vi "Plot Editor_Store to Plot.vi"(7 "XYGraph in":refnum<vi>, 8 "Error In":errorcluster, 11 "Plot Editor Internal Data":T1) -> (0 "Error Out":errorcluster, 3 "Plot Editor Internal Data (dup)":T1)   [LabVIEW 2021, in "Plot Editor.lvlib"]
uses:
  Plot Editor.lvlib
  Plot Editor Internal Variables.ctl
  XY Graph/XY Graph Plot Properties.ctl
  XY Graph/XY Graph Add-Ons.lvlib
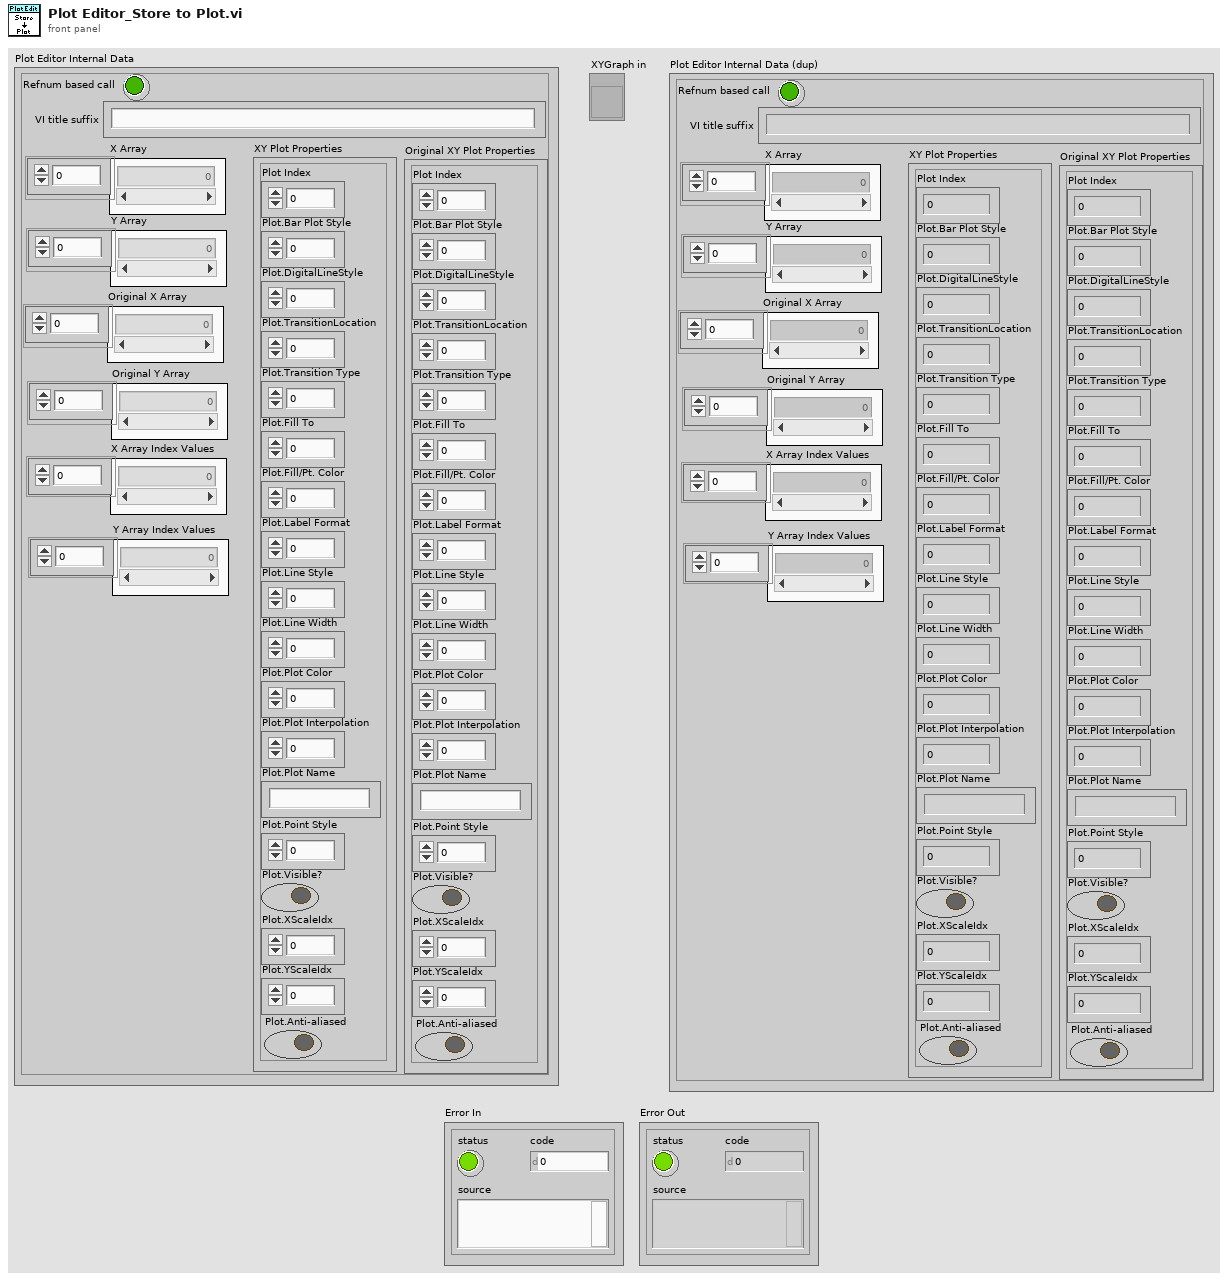
[diagram p1: front panel]
types:
  T1 = typedef "Plot Editor.lvlib/Plot Editor Internal Variables.ctl" = cluster{"X Array":dbl[], "Y Array":dbl[], "XY Plot Properties":T2, "X Array Index Values":u32[], "Y Array Index Values":u32[], "Original XY Plot Properties":T2, "Original X Array":dbl[], "Original Y Array":dbl[], "VI title suffix":string, "Refnum based call":bool}
  T2 = typedef "XY Graph Add-Ons.lvlib/XY Graph Plot Properties.ctl" = cluster{"Plot Index":i32, "Plot.Bar Plot Style":u8, "Plot.DigitalLineStyle":u8, "Plot.TransitionLocation":u8, "Plot.Transition Type":u8, "Plot.Fill To":i16, "Plot.Fill/Pt. Color":u32, "Plot.Label Format":u8, "Plot.Line Style":u8, "Plot.Line Width":u8, "Plot.Plot Color":u32, "Plot.Plot Interpolation":u8, "Plot.Plot Name":string, "Plot.Point Style":u8, "Plot.Visible?":bool, "Plot.XScaleIdx":u32, "Plot.YScaleIdx":u32, "Plot.Anti-aliased":bool}
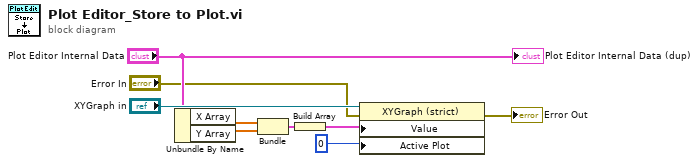
[diagram p0: block diagram]
diagram:
  n1 = Unbundle By Name("Plot Editor Internal Data") -> ("X Array"=w7:dbl[], "Y Array"=w8:dbl[])
  n2 = Bundle("X Array"=w7, "Y Array"=w8) -> (w5:cluster{"X Array":dbl[], "Y Array":dbl[]})  [unwired: 1 in]
  n3 = Build Array(w5) -> (w6:cluster{"X Array":dbl[], "Y Array":dbl[]}[])
  n4 = property on="Property Node" class="XYGraph (strict)"(reference="XYGraph in", error in="Error In", "Value"=w6, "Active Plot"=u32 0) -> (error out=→"Error Out":errorcluster)  [unwired: 1 out]
  "Plot Editor Internal Data (dup)" <- "Plot Editor Internal Data"
